vi "Calculate Money Left.vi"(8 "error in (no error)":errorcluster, 11 "Database in":refnum<class "Database.lvclass">) -> (0 "error out":errorcluster, 3 "Database out":refnum<class "Database.lvclass">)   [LabVIEW 2018]
uses:
  Database.lvclass
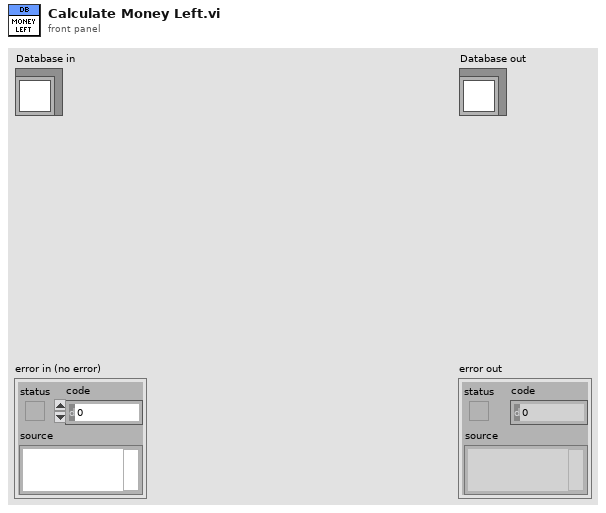
[diagram p1: front panel]
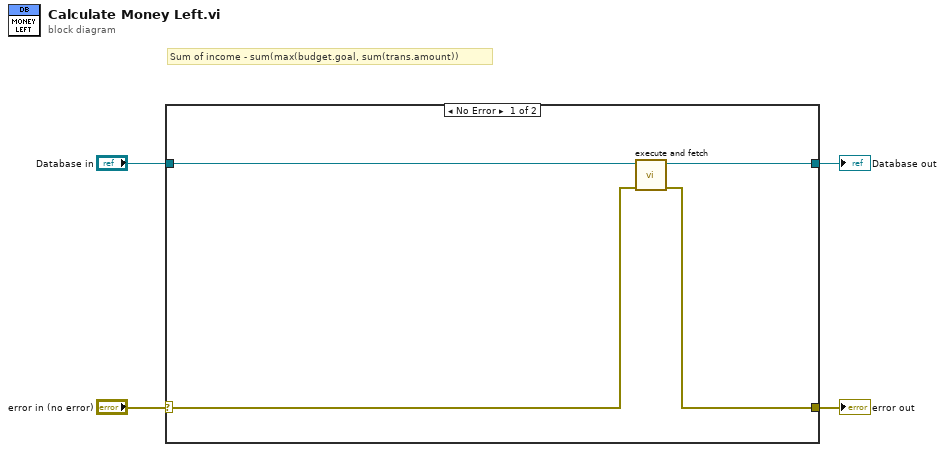
[diagram p0: block diagram]
diagram:
  # "Sum of income - sum(max(budget.goal, sum(trans.amount))"
  n1 = case shown="No Error" "error in (no error)" {
    selector: "error in (no error)" -> [w5 w10]
    tunnel: [w6 w10] -> w3
    tunnel: [w7 w9] -> w1
    tunnel: "Database in" -> [w8 w9]
    frame No Error {
      n2 = call "execute and fetch.vi"("error in (no error)"=w5, "Database in"=w8) -> ("error out"=w6:errorcluster, "Database out"=w7:refnum<class "Database.lvclass">)  [unwired: 6 in, 2 out]
    }
    frame Error {
    }
  }
  "error out" <- w3
  "Database out" <- w1
